vi "evenOdd.vi"(1 "number":dbl) -> (0 "odd/even":bool)   [LabVIEW 2015]
panel:
  # "true if even"
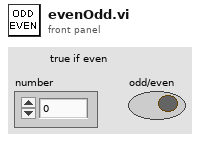
[diagram p1: front panel]
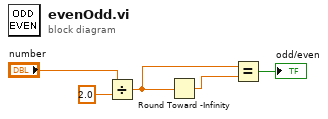
[diagram p0: block diagram]
diagram:
  n1 = Divide(x="number", y=2.0) -> (x/y=w4:dbl)
  n2 = Round Toward -Infinity(1:w4) -> (0:w3:dbl)
  n3 = Equal?(x=w4, y=w3) -> (x = y?=→"odd/even":bool)
